vi "SubCarrModulate.vi"(8 "error in (no error)":errorcluster, 11 "ISO 14443 A UP in":refnum<class "ISO 14443 A UP.lvclass">) -> (0 "error out":errorcluster, 3 "ISO 14443 A UP out":refnum<class "ISO 14443 A UP.lvclass">)   [LabVIEW 2019, in "ISO 14443 A UP.lvclass"]
uses:
  ISO 14443 A UP.lvclass
  TypeDef/Store.ctl
  ISO 14443 A UP.lvclass/ISO 14443 A UP.ctl
  RFID system.lvclass
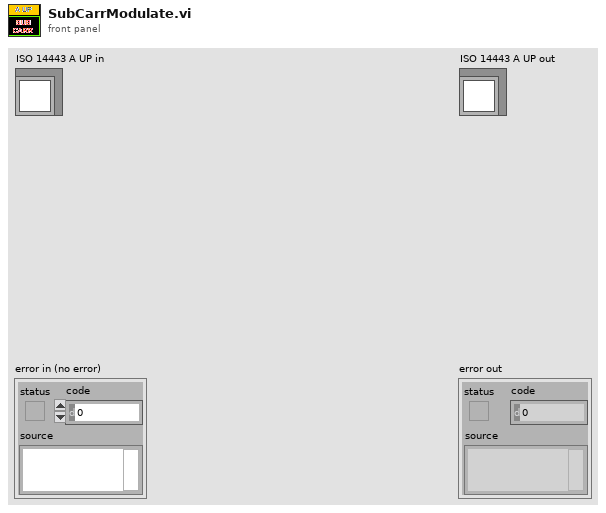
[diagram p1: front panel]
types:
  T1 = typedef "Store.ctl" = enum16{"envelope", "noise", "demSubCar", "CH_frame", "Decode", "demodulate", "in", "out", "sum", "subCarrier", "frame", "command", "encode", "modulate", "encode_UP", "modulate_up", "demod_up", "envelop_up", "sum_up", "out_up", "in_up"}
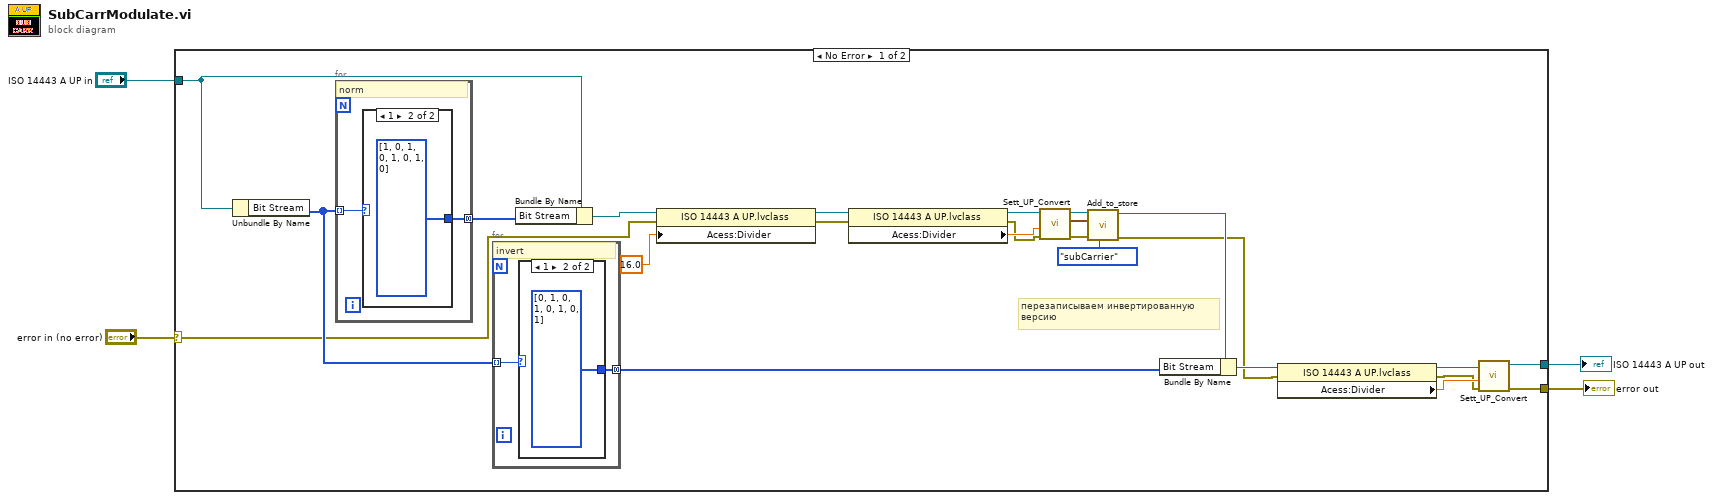
[diagram p0: block diagram]
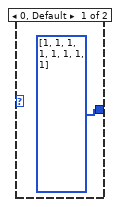
[diagram p2: hidden frame]
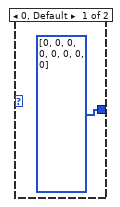
[diagram p3: hidden frame]
diagram:
  n1 = case shown="No Error" "error in (no error)" {
    selector: "error in (no error)" -> [w11 w37]
    tunnel: [w16 w37] -> w3
    tunnel: "ISO 14443 A UP in" -> [w27 w38]
    tunnel: [w17 w38] -> w1
    frame No Error {
      # "перезаписываем инвертированную\nверсию"
      n2 = Unbundle By Name(w27) -> ("Bit Stream"=w28:u8[])
      n3 = for {
        tunnel: w28 -> [w34] mode=indexing
        tunnel: [w33] -> w26 mode=concatenating
        # "norm"
        n4 = case shown="1" w34 {
          tunnel: [u8[] [0, 0, 0, 0, 0, 0, 0, 0] ("output array") u8[] [1, 0, 1, 0, 1, 0, 1, 0] ("output array")] -> w33
          frame 0, Default {
          }
          frame 1 {
          }
        }
      }
      n5 = for {
        tunnel: w28 -> [w29] mode=indexing
        tunnel: [w30] -> w19 mode=concatenating
        # "invert"
        n6 = case shown="1" w29 {
          tunnel: [u8[] [1, 1, 1, 1, 1, 1, 1, 1] ("output array") u8[] [0, 1, 0, 1, 0, 1, 0, 1] ("output array")] -> w30
          frame 0, Default {
          }
          frame 1 {
          }
        }
      }
      n7 = Bundle By Name(cluster=w27, "Bit Stream"=w26) -> (w25:refnum<class "ISO 14443 A UP.lvclass">)
      n8 = property class="ISO 14443 A UP.lvclass"(reference=w25, error in=w11, "Acess:Divider"=16.0 ("Divider(1)")) -> (reference out=w12:refnum<class "ISO 14443 A UP.lvclass">, error out=w10:errorcluster)
      n9 = property class="ISO 14443 A UP.lvclass"(reference=w12, error in=w10) -> (reference out=w15:refnum<class "ISO 14443 A UP.lvclass">, error out=w13:errorcluster, "Acess:Divider"=w14:dbl)
      n10 = call-dynamic "Sett_UP_Convert.vi"("error in (no error)"=w13, "Divider(1)"=w14, "ISO 14443 A UP in"=w15) -> ("error out"=w22:errorcluster, "Waveform"=w23:waveform(dbl), "ISO 14443 A UP out"=w24:refnum<class "ISO 14443 A UP.lvclass">)  [unwired: 6 in]
      n11 = call "Add_to_store.vi"("Store"=Store."subCarrier", "error in (no error)"=w22, "Waveform"=w23, "RFID system in"=w24) -> ("error out"=w6:errorcluster, "RFID system out"=w20:refnum<class "ISO 14443 A UP.lvclass">)  [unwired: 6 in]
      n12 = Bundle By Name(cluster=w20, "Bit Stream"=w19) -> (w18:refnum<class "ISO 14443 A UP.lvclass">)
      n13 = property class="ISO 14443 A UP.lvclass"(reference=w18, error in=w6) -> (reference out=w8:refnum<class "ISO 14443 A UP.lvclass">, error out=w5:errorcluster, "Acess:Divider"=w7:dbl)
      n14 = call-dynamic "Sett_UP_Convert.vi"("error in (no error)"=w5, "Divider(1)"=w7, "ISO 14443 A UP in"=w8) -> ("error out"=w16:errorcluster, "ISO 14443 A UP out"=w17:refnum<class "ISO 14443 A UP.lvclass">)  [unwired: 6 in, 1 out]
    }
    frame Error {
    }
  }
  "error out" <- w3
  "ISO 14443 A UP out" <- w1
